vi "Multiplexer 4 to 1.vi"() -> ()   [LabVIEW 2020]
panel:
  out "F":bool
  in  "S0":bool
  in  "S1":bool
  in  "I3":bool
  in  "I2":bool
  in  "I1":bool
  in  "I0":bool
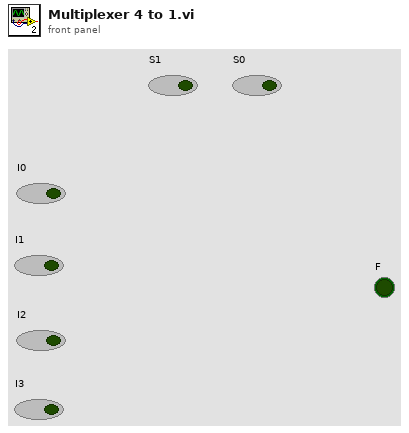
[diagram p1: front panel]
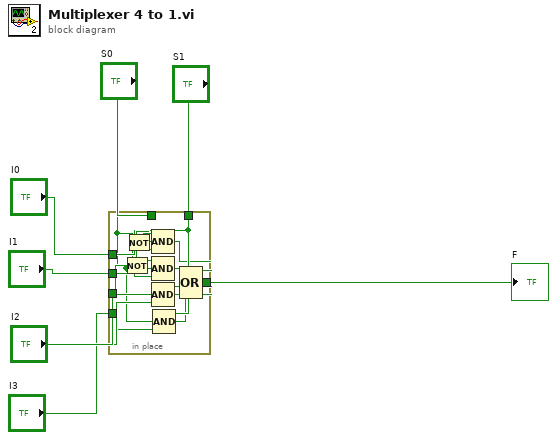
[diagram p0: block diagram]
diagram:
  n1 = in-place {
    in-place-border: "I0" -> [w20]
    in-place-border: "I1" -> [w18]
    in-place-border: "I2" -> [w16]
    in-place-border: "S1" -> [w15]
    in-place-border: "S0" -> [w14]
    in-place-border: "I3" -> [w13]
    in-place-border: [w8] -> w1
    n2 = Not(x=w14) -> (.not. x?=w17:bool)
    n3 = Not(x=w15) -> (.not. x?=w19:bool)
    n4 = Compound Arithmetic op=AND(w19, w17, w20) -> (w12:bool)
    n5 = Compound Arithmetic op=AND(w19, w14, w18) -> (w11:bool)
    n6 = Compound Arithmetic op=AND(w15, w17, w16) -> (w10:bool)
    n7 = Compound Arithmetic op=AND(w15, w14, w13) -> (w9:bool)
    n8 = Compound Arithmetic op=OR(w12, w11, w10, w9) -> (w8:bool)
  }
  "F" <- w1
